vi "DAQ_Stop_Clear_Tasks.vi"(8 "error in":errorcluster caption="entrée d'erreur", 11 "Cluster tasks":T1) -> (0 "sortie d'erreur":errorcluster)   [LabVIEW 2026]
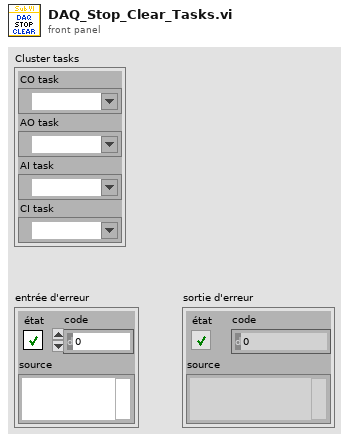
[diagram p1: front panel]
types:
  T1 = cluster{"CO task":refnum<k21>, "AO task":refnum<k21>, "AI task":refnum<k21>, "CI task":refnum<k21>}
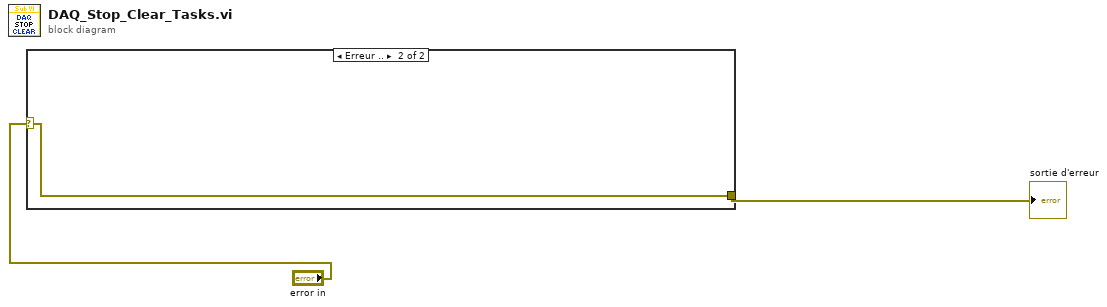
[diagram p0: block diagram]
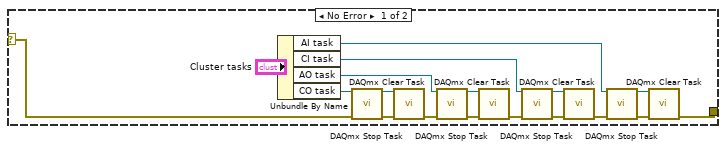
[diagram p2: hidden frame]
diagram:
  n1 = case shown="Erreur .." "error in" {
    selector: "error in" -> [w3 w21]
    tunnel: [w15 w21] -> w2
    frame No Error {
      n2 = Unbundle By Name("Cluster tasks") -> ("AI task"=w19:refnum<k21>, "CI task"=w18:refnum<k21>, "AO task"=w17:refnum<k21>, "CO task"=w16:refnum<k21>)
      n3 = call <vilib>:"DAQmx Stop Task.vi"("task/channels in"=w16, "error in"=w3) -> ("task out"=w4:refnum<k21>, "error out"=w5:errorcluster)  [unwired: 12 in]
      n4 = call <vilib>:"DAQmx Clear Task.vi"("task in"=w4, "error in"=w5) -> ("error out"=w12:errorcluster)  [unwired: 13 in]
      n5 = call <vilib>:"DAQmx Stop Task.vi"("task/channels in"=w17, "error in"=w12) -> ("task out"=w7:refnum<k21>, "error out"=w6:errorcluster)  [unwired: 12 in]
      n6 = call <vilib>:"DAQmx Clear Task.vi"("task in"=w7, "error in"=w6) -> ("error out"=w13:errorcluster)  [unwired: 13 in]
      n7 = call <vilib>:"DAQmx Stop Task.vi"("task/channels in"=w18, "error in"=w13) -> ("task out"=w8:refnum<k21>, "error out"=w9:errorcluster)  [unwired: 12 in]
      n8 = call <vilib>:"DAQmx Clear Task.vi"("task in"=w8, "error in"=w9) -> ("error out"=w14:errorcluster)  [unwired: 13 in]
      n9 = call <vilib>:"DAQmx Stop Task.vi"("task/channels in"=w19, "error in"=w14) -> ("task out"=w11:refnum<k21>, "error out"=w10:errorcluster)  [unwired: 12 in]
      n10 = call <vilib>:"DAQmx Clear Task.vi"("task in"=w11, "error in"=w10) -> ("error out"=w15:errorcluster)  [unwired: 13 in]
    }
    frame Error {
    }
  }
  "sortie d'erreur" <- w2
